vi "gm_sqlite_write_measvalues.vi"(8 "error in (no error)":errorcluster, 10 "Database File":string, 11 "Output - Cluster gas":T1 {"GM TS-2[°C]" format="%.2g"; "GM TS-1 [°C]" format="%.2g"; "GM DS-1 [bar]" format="%.4g"; "GM DS-2 [bar]" format="%.4g"; "GA1 h2 [%]" format="%.2g"; "GA1 co2 [%]" format="%.2g"; "GA1 ch4 [%]" format="%.2g"}) -> (0 "error out":errorcluster)   [LabVIEW 2011]
uses:
  Output - Cluster gas.ctl
  gas_values.ctl
panel:
  # "qualitätsmessung"
  # "quantitätsmessung"
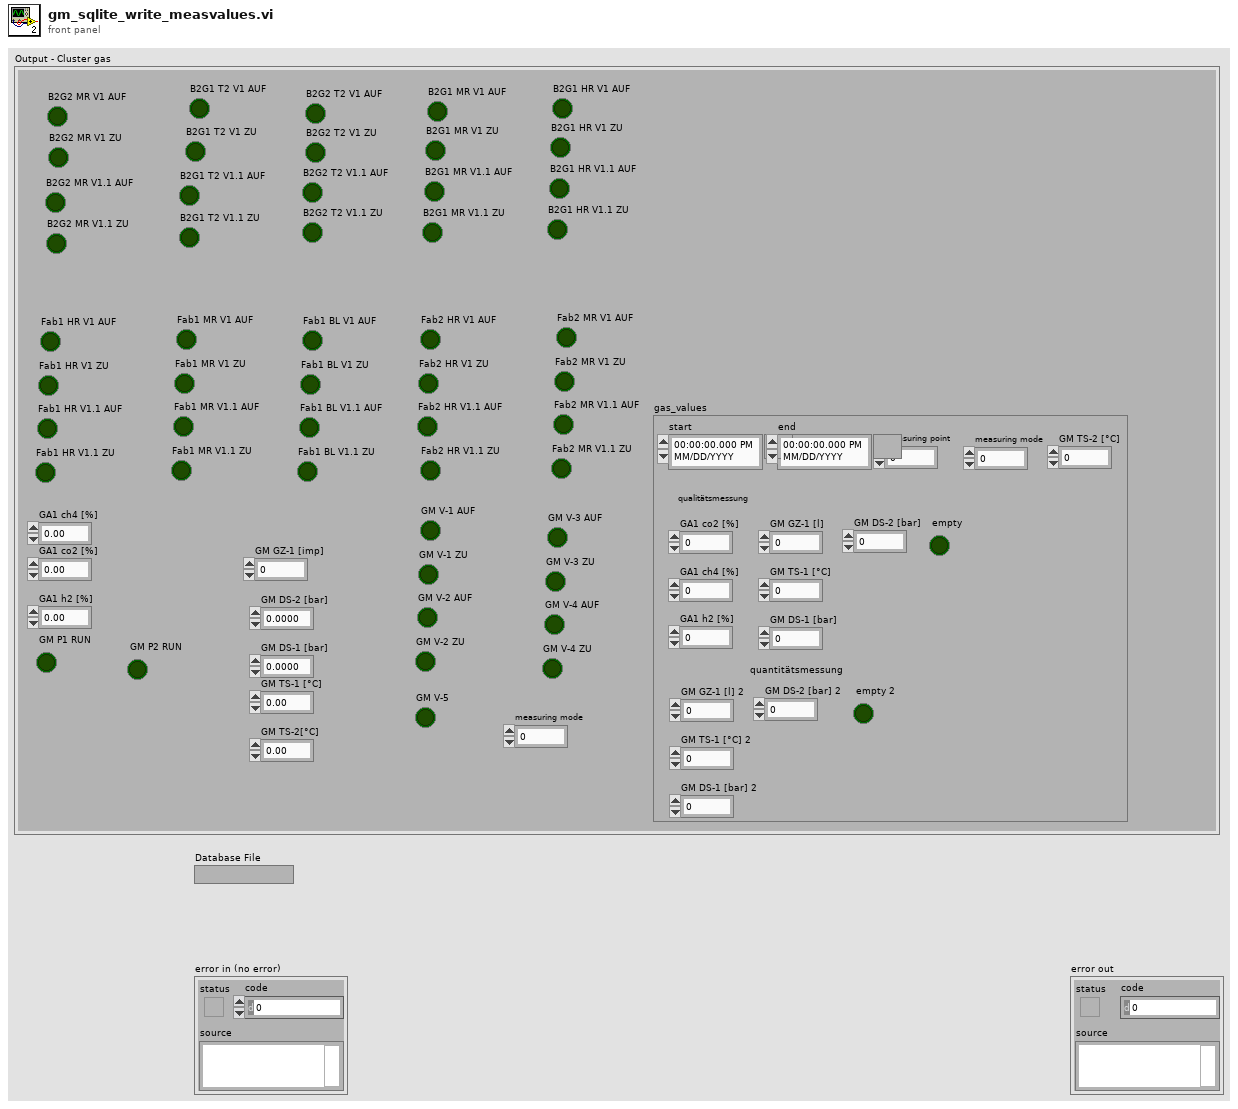
[diagram p1: front panel]
types:
  T1 = typedef "Output - Cluster gas.ctl" = cluster{"B2G2 MR V1.1 AUF":bool, "B2G2 MR V1.1 ZU":bool, "B2G2 MR V1 AUF":bool, "B2G2 MR V1 ZU":bool, "B2G1 T2 V1 AUF":bool, "B2G1 T2 V1 ZU":bool, "B2G1 T2 V1.1 AUF":bool, "B2G1 T2 V1.1 ZU":bool, "B2G2 T2 V1 AUF":bool, "B2G2 T2 V1 ZU":bool, "B2G2 T2 V1.1 ZU":bool, "B2G2 T2 V1.1 AUF":bool, "B2G1 MR V1 AUF":bool, "B2G1 MR V1 ZU":bool, "B2G1 MR V1.1 AUF":bool, "B2G1 MR V1.1 ZU":bool, "B2G1 HR V1 AUF":bool, "B2G1 HR V1 ZU":bool, "B2G1 HR V1.1 AUF":bool, "B2G1 HR V1.1 ZU":bool, "Fab1 HR V1 AUF":bool, "Fab1 HR V1 ZU":bool, "Fab1 HR V1.1 AUF":bool, "Fab1 HR V1.1 ZU":bool, "Fab1 MR V1 AUF":bool, "Fab1 MR V1 ZU":bool, "Fab1 MR V1.1 AUF":bool, "Fab1 MR V1.1 ZU":bool, "Fab1 BL V1 AUF":bool, "Fab1 BL V1 ZU":bool, "Fab1 BL V1.1 AUF":bool, "Fab1 BL V1.1 ZU":bool, "Fab2 HR V1 AUF":bool, "Fab2 HR V1 ZU":bool, "Fab2 HR V1.1 AUF":bool, "Fab2 HR V1.1 ZU":bool, "Fab2 MR V1 AUF":bool, "Fab2 MR V1 ZU":bool, "Fab2 MR V1.1 AUF":bool, "Fab2 MR V1.1 ZU":bool, "GA1 ch4 [%]":dbl, "GA1 co2 [%]":dbl, "GA1 h2 [%]":dbl, "GM P1 RUN":bool, "GM V-1 AUF":bool, "GM V-1 ZU":bool, "GM V-2 AUF":bool, "GM V-2 ZU":bool, "GM V-3 AUF":bool, "GM V-3 ZU":bool, "GM V-4 AUF":bool, "GM V-4 ZU":bool, "GM P2 RUN":bool, "GM GZ-1 [imp]":u32, "GM DS-2 [bar]":dbl, "GM DS-1 [bar]":dbl, "GM TS-1 [°C]":dbl, "GM TS-2[°C]":dbl, "gas_values":T2, "measuring mode":u8, "GM V-5":bool}
  T2 = typedef "gas_values.ctl" = cluster{"start":timestamp, "GM DS-2 [bar]":dbl, "GA1 ch4 [%]":dbl, "GA1 co2 [%]":dbl, "GA1 h2 [%]":dbl, "GM DS-1 [bar]":dbl, "GM TS-1 [°C]":dbl, "GM TS-2 [°C]":dbl, "GM GZ-1 [l]":dbl, "measuring point":u8, "end":timestamp, "empty":bool, "GM GZ-1 [l] 2":dbl, "GM TS-1 [°C] 2":dbl, "GM DS-1 [bar] 2":dbl, "GM DS-2 [bar] 2":dbl, "empty 2":bool, "measuring mode":u8}
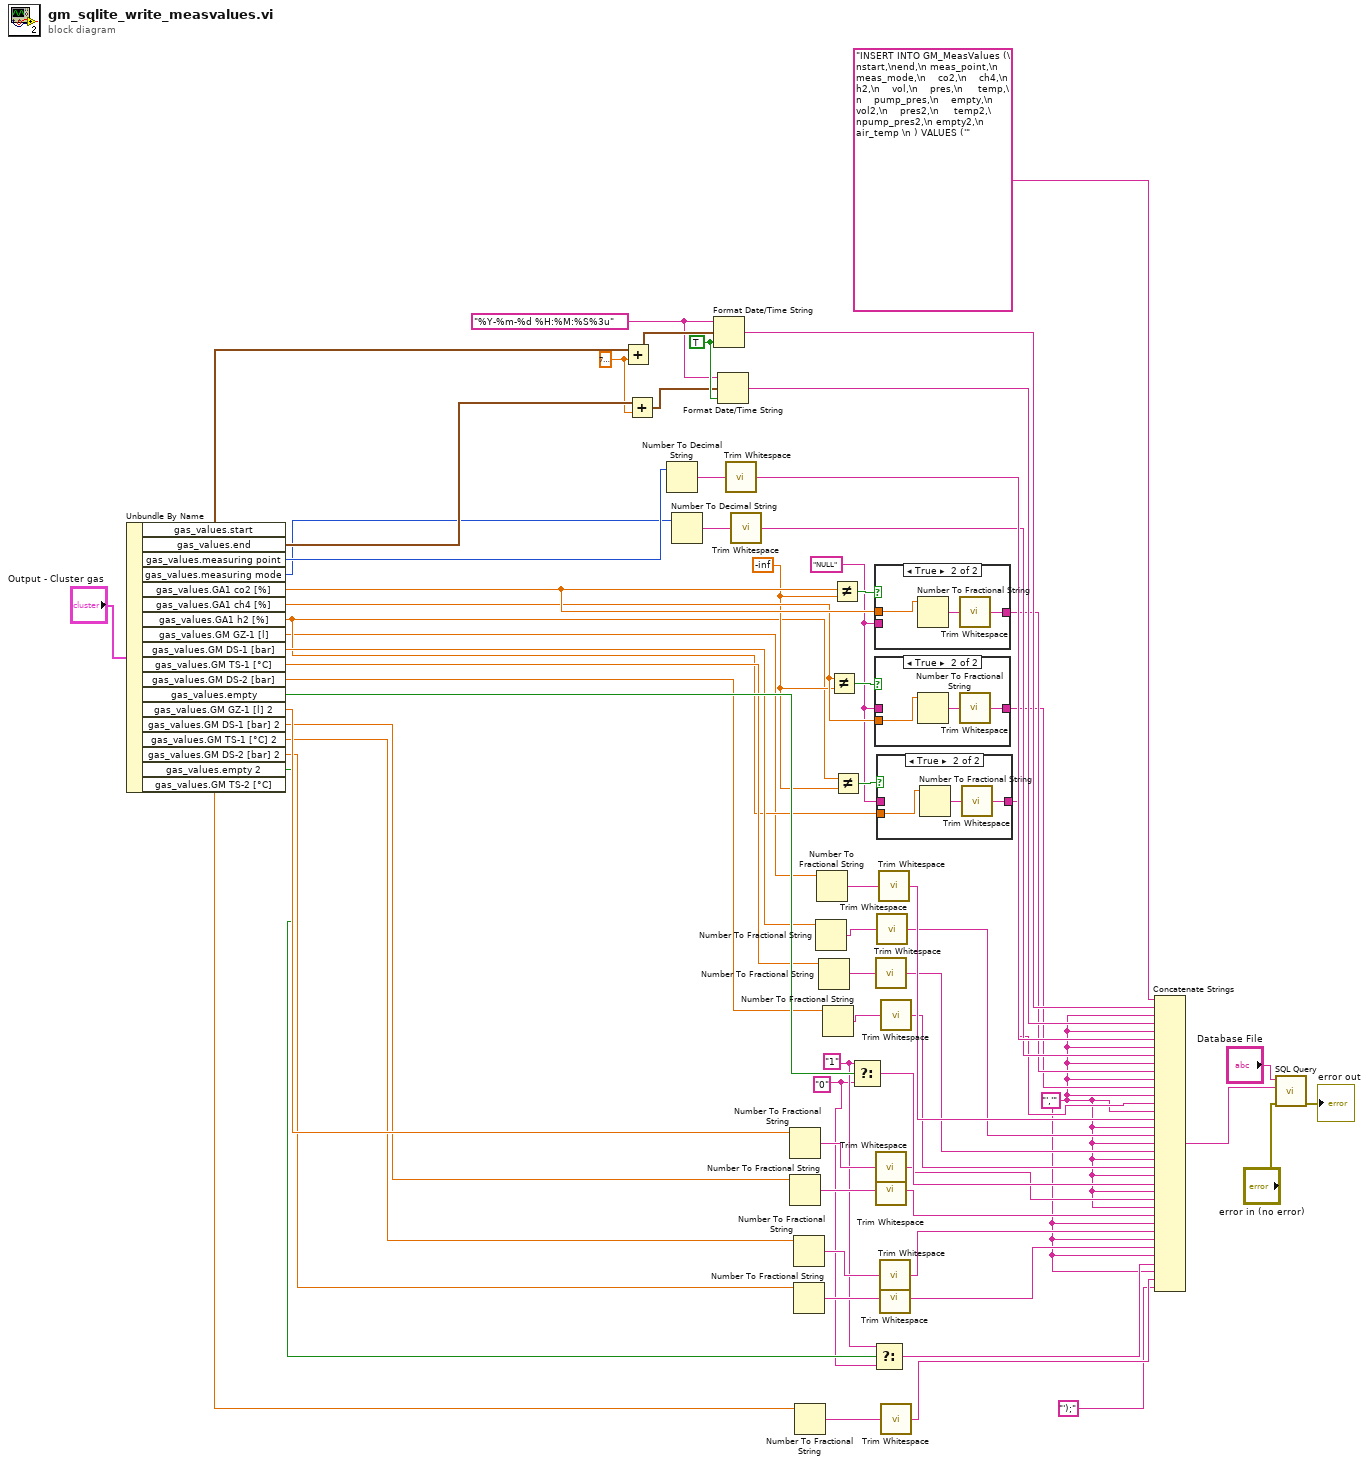
[diagram p0: block diagram]
diagram:
  w39 = dbl[unit] 7200.0 ("y")
  w43 = TRUE ("UTC format")
  w46 = "NULL" ("trimmed string")
  w49 = -inf ("y")
  w42 = "%Y-%m-%d %H:%M:%S%3u" ("time format string (%c)")
  w5 = "','" ("string")
  w1 = "0"
  w2 = "1"
  n1 = Unbundle By Name("Output - Cluster gas") -> ("gas_values.start"=w44:timestamp, "gas_values.end"=w41:timestamp, "gas_values.measuring point"=w38:u8, "gas_values.measuring mode"=w35:u8, "gas_values.GA1 co2 [%]"=w53:dbl, "gas_values.GA1 ch4 [%]"=w50:dbl, "gas_values.GA1 h2 [%]"=w47:dbl, "gas_values.GM GZ-1 [l]"=w32:dbl, "gas_values.GM DS-1 [bar]"=w60:dbl, "gas_values.GM TS-1 [°C]"=w58:dbl, "gas_values.GM DS-2 [bar]"=w55:dbl, "gas_values.empty"=w61:bool, "gas_values.GM GZ-1 [l] 2"=w34:dbl, "gas_values.GM DS-1 [bar] 2"=w29:dbl, "gas_values.GM TS-1 [°C] 2"=w28:dbl, "gas_values.GM DS-2 [bar] 2"=w27:dbl, "gas_values.empty 2"=w26:bool, "gas_values.GM TS-2 [°C]"=w24:dbl)
  n2 = Add(x=w44, y=w39) -> (x+y=w45:timestamp)
  n3 = Add(x=w41, y=w39) -> (x+y=w40:timestamp)
  n4 = Number To Decimal String(number=w38) -> (decimal integer string=w37:string)  [unwired: 1 in]
  n5 = Number To Decimal String(number=w35) -> (decimal integer string=w36:string)  [unwired: 1 in]
  n6 = Format Date/Time String(time format string (%c)=w42, seconds (now)=w45, UTC format=w43) -> (date/time string=w22:string)
  n7 = Format Date/Time String(time format string (%c)=w42, seconds (now)=w40, UTC format=w43) -> (date/time string=w21:string)
  n8 = call <vilib>:"Trim Whitespace.vi"("string"=w37) -> ("trimmed string"=w20:string)  [unwired: 1 in]
  n9 = call <vilib>:"Trim Whitespace.vi"("string"=w36) -> ("trimmed string"=w19:string)  [unwired: 1 in]
  n10 = Number To Fractional String(number=w34) -> (F-format string=w63:string)  [unwired: 3 in]
  n11 = Number To Fractional String(number=w29) -> (F-format string=w56:string)  [unwired: 3 in]
  n12 = Number To Fractional String(number=w28) -> (F-format string=w30:string)  [unwired: 3 in]
  n13 = Number To Fractional String(number=w27) -> (F-format string=w31:string)  [unwired: 3 in]
  n14 = Number To Fractional String(number=w24) -> (F-format string=w25:string)  [unwired: 3 in]
  n15 = Number To Fractional String(number=w60) -> (F-format string=w59:string)  [unwired: 3 in]
  n16 = Number To Fractional String(number=w32) -> (F-format string=w33:string)  [unwired: 3 in]
  n17 = Number To Fractional String(number=w58) -> (F-format string=w57:string)  [unwired: 3 in]
  n18 = Number To Fractional String(number=w55) -> (F-format string=w54:string)  [unwired: 3 in]
  n19 = Not Equal?(x=w50, y=w49) -> (x != y?=w51:bool)
  n20 = Not Equal?(x=w53, y=w49) -> (x != y?=w52:bool)
  n21 = Not Equal?(x=w47, y=w49) -> (x != y?=w48:bool)
  n22 = Select(t=w2, s=w61, f=w1) -> (s? t:f=w11:string)
  n23 = Select(t=w2, s=w26, f=w1) -> (s? t:f=w6:string)
  n24 = case shown="True" w52 {
    tunnel: w53 -> [_ w70]
    tunnel: [w68 w69] -> w18
    tunnel: w46 -> [w68 _]
    frame False {
    }
    frame True {
      n25 = Number To Fractional String(number=w70) -> (F-format string=w71:string)  [unwired: 3 in]
      n26 = call <vilib>:"Trim Whitespace.vi"("string"=w71) -> ("trimmed string"=w69:string)  [unwired: 1 in]
    }
  }
  n27 = case shown="True" w51 {
    tunnel: w50 -> [_ w74]
    tunnel: [w72 w73] -> w17
    tunnel: w46 -> [w72 _]
    frame False {
    }
    frame True {
      n28 = Number To Fractional String(number=w74) -> (F-format string=w75:string)  [unwired: 3 in]
      n29 = call <vilib>:"Trim Whitespace.vi"("string"=w75) -> ("trimmed string"=w73:string)  [unwired: 1 in]
    }
  }
  n30 = call <vilib>:"Trim Whitespace.vi"("string"=w57) -> ("trimmed string"=w13:string)  [unwired: 1 in]
  n31 = call <vilib>:"Trim Whitespace.vi"("string"=w63) -> ("trimmed string"=w10:string)  [unwired: 1 in]
  n32 = call <vilib>:"Trim Whitespace.vi"("string"=w56) -> ("trimmed string"=w9:string)  [unwired: 1 in]
  n33 = case shown="True" w48 {
    tunnel: [w76 w78] -> w16
    tunnel: w47 -> [_ w77]
    tunnel: w46 -> [w76 _]
    frame False {
    }
    frame True {
      n34 = Number To Fractional String(number=w77) -> (F-format string=w79:string)  [unwired: 3 in]
      n35 = call <vilib>:"Trim Whitespace.vi"("string"=w79) -> ("trimmed string"=w78:string)  [unwired: 1 in]
    }
  }
  n36 = call <vilib>:"Trim Whitespace.vi"("string"=w59) -> ("trimmed string"=w14:string)  [unwired: 1 in]
  n37 = call <vilib>:"Trim Whitespace.vi"("string"=w33) -> ("trimmed string"=w15:string)  [unwired: 1 in]
  n38 = call <vilib>:"Trim Whitespace.vi"("string"=w30) -> ("trimmed string"=w8:string)  [unwired: 1 in]
  n39 = call <vilib>:"Trim Whitespace.vi"("string"=w31) -> ("trimmed string"=w7:string)  [unwired: 1 in]
  n40 = call <vilib>:"Trim Whitespace.vi"("string"=w54) -> ("trimmed string"=w12:string)  [unwired: 1 in]
  n41 = call <vilib>:"Trim Whitespace.vi"("string"=w25) -> ("trimmed string"=w4:string)  [unwired: 1 in]
  n42 = Concatenate Strings("INSERT INTO GM_MeasValues (\nstart,\nend,\n meas_point,\n  meas_mode,\n    co2,\n    ch4,\n    h2,\n    vol,\n    pres,\n     temp,\n    pump_pres,\n    empty,\n  vol2,\n    pres2,\n     temp2,\npump_pres2,\n empty2,\n    air_temp \n ) VALUES ('" ("SQL Query"), w22, w5, w21, w5, w20, w5, w19, w5, w18, w5, w17, w5, w16, w5, w15, w5, w14, w5, w13, w5, w12, w5, w11, w5, w10, w5, w9, w5, w8, w5, w7, w5, w6, w5, w4, "');" ("string")) -> (w62:string)
  n43 = call "SQL Query.vi"("error in (no error)"="error in (no error)", "SQL Query"=w62, "Database File"="Database File") -> ("error out"=→"error out":errorcluster)  [unwired: 6 in, 2 out]
